vi "Server Thread Send Message.vi"(1 "error in":errorcluster, 2 "Vision Message":cluster{"Type":string, "Message":string}, 3 "Server Thread":cluster{"connection ID":refnum<k5>}) -> (0 "error out":errorcluster)   [LabVIEW 2016]
uses:
  Messages/Heartbeat/Heartbeat Message to JSON.vi
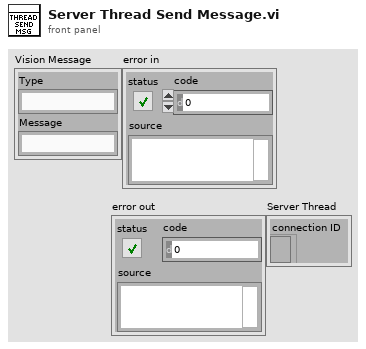
[diagram p1: front panel]
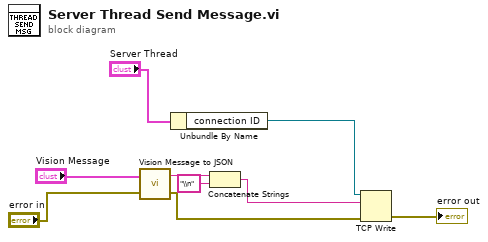
[diagram p0: block diagram]
diagram:
  n1 = call-poly "Vision Message to JSON.vi"("error in"="error in", "Heartbeat Message"="Vision Message") -> ("error out"=w2:errorcluster, "JSON string"=w7:string)
  n2 = Unbundle By Name("Server Thread") -> ("connection ID"=w4:refnum<k5>)
  n3 = Concatenate Strings(w7, "\\n" ("string")) -> (w3:string)
  n4 = TCP Write(connection ID=w4, data in=w3, error in (no error)=w2) -> (error out=→"error out":errorcluster)  [unwired: 1 in, 2 out]
